vi "move item between listboxes.vi"(8 "error in":errorcluster, 10 "target":refnum<vi>, 11 "source":refnum<vi>) -> (0 "error out":errorcluster, 2 "new target":string[](array[string]), 3 "new source":string[](array[string]))   [LabVIEW 2013]
panel:
  out "moved item":string
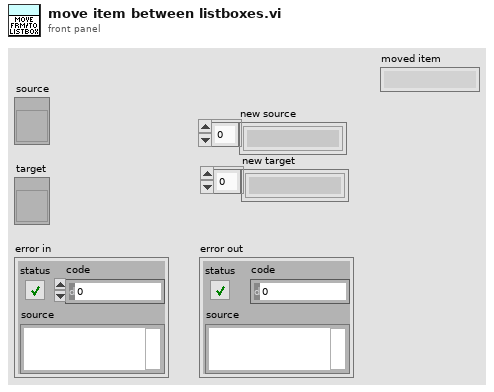
[diagram p1: front panel]
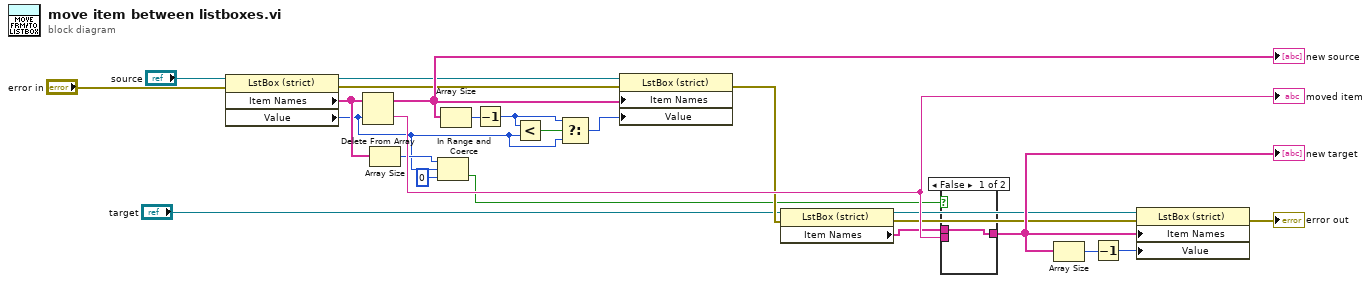
[diagram p0: block diagram]
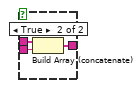
[diagram p2: hidden frame]
diagram:
  n1 = property class="LstBox (strict)"(reference="source", error in="error in") -> (reference out=w7:refnum<vi>, error out=w6:errorcluster, "Item Names"=w5:string[], "Value"=w3:i32)
  n2 = Delete From Array(array=w5, index=w3) -> (deleted portion=w21:string, array with subset deleted=w8:string[])  [unwired: 1 in]
  "new source" <- w8
  "moved item" <- w21
  n3 = Array Size(array=w5) -> (size(s)=w4:i32)
  n4 = In Range and Coerce(upper limit=w4, x=w3, lower limit=0) -> (In Range?=w1:bool)  [unwired: 1 out]
  n5 = Array Size(array=w8) -> (size(s)=w9:i32)
  n6 = Decrement(x=w9) -> (x-1=w11:i32)
  n7 = Less?(x=w11, y=w3) -> (x < y?=w10:bool)
  n8 = Select(t=w11, s=w10, f=w3) -> (s? t:f=w12:i32)
  n9 = property class="LstBox (strict)"(reference=w7, error in=w6, "Item Names"=w8, "Value"=w12) -> (error out=w17:errorcluster)  [unwired: 1 out]
  n10 = property class="LstBox (strict)"(reference="target", error in=w17) -> (reference out=w14:refnum<vi>, error out=w15:errorcluster, "Item Names"=w20:string[])
  n11 = case shown="False" w1 {
    tunnel: [w25 w28] -> w22
    tunnel: w21 -> [_ w27]
    tunnel: w20 -> [w25 w26]
    frame False {
    }
    frame True {
      n12 = Build Array (concatenate)(w26, w27) -> (w28:string[])
    }
  }
  "new target" <- w22
  n13 = Array Size(array=w22) -> (size(s)=w24:i32)
  n14 = Decrement(x=w24) -> (x-1=w23:i32)
  n15 = property class="LstBox (strict)"(reference=w14, error in=w15, "Item Names"=w22, "Value"=w23) -> (error out=→"error out":errorcluster)  [unwired: 1 out]
